vi "simx Set Object Parent.vi"(6 "operationMode":i32, 7 "keepInPlace":u8, 8 "error in (no error)":errorcluster, 9 "parentObject":i32, 10 "objectHandle":i32, 11 "clientID":i32) -> (0 "error out":errorcluster, 3 "function return":i32)   [LabVIEW 2019, in "PXL_V-REP.lvlib"]
doc: "EXTAPI_DLLEXPORT simxInt simxSetObjectParent(simxInt clientID,simxInt objectHandle,simxInt parentObject,simxUChar keepInPlace,simxInt operationMode);"
uses:
  PXL_V-REP.lvlib
  <userlib>/V-REP/remoteApi.dll
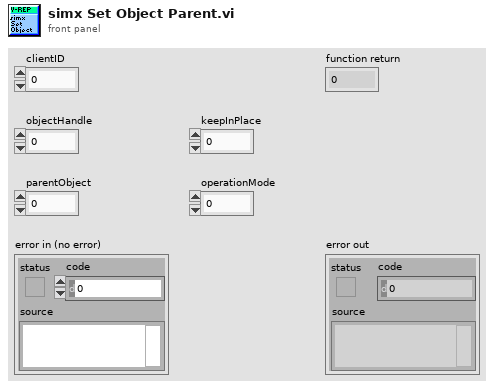
[diagram p1: front panel]
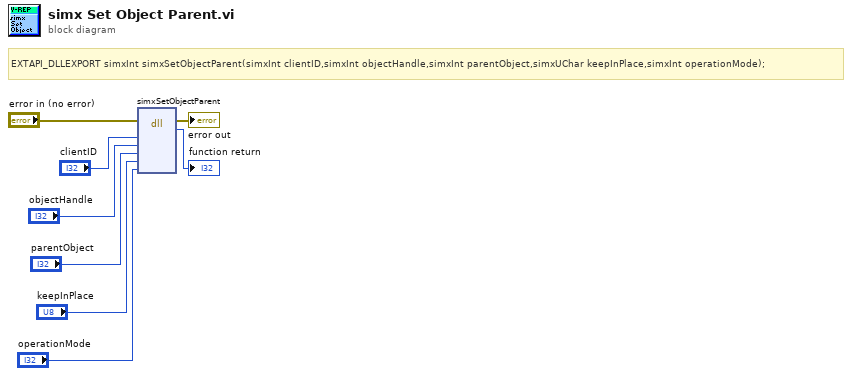
[diagram p0: block diagram]
diagram:
  # "EXTAPI_DLLEXPORT simxInt simxSetObjectParent(simxInt clientID,simxInt objectHandle,simxInt parentObject,simxUChar keepInPlace,simxInt operationMode);"
  n1 = dll-call lib="C:/Program Files (x86)/National Instruments/LabVIEW 2019/user.lib/V-REP/remoteApi.*" fn="simxSetObjectParent"(error in="error in (no error)", "clientID"="clientID", "objectHandle"="objectHandle", "parentObject"="parentObject", "keepInPlace"="keepInPlace", "operationMode"="operationMode") -> (error out=→"error out":errorcluster, →"function return":i32)  [unwired: 7 in, 1 out]
